vi "Get KB Name.vi"(11 "KB Name":string) -> (3 "KB Name":string)   [LabVIEW 2023, in "LabVIEW RAG.lvlib"]
uses:
  LabVIEW RAG.lvlib
  AI RAG Globals.vi
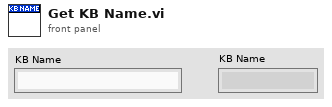
[diagram p1: front panel]
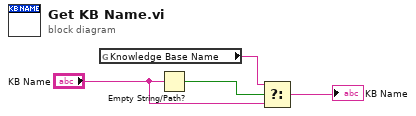
[diagram p0: block diagram]
diagram:
  n1 = global read "AI RAG Globals.vi" "Knowledge Base Name"() -> (w4:string)
  n2 = Empty String/Path?(string/path="KB Name") -> (empty?=w3:bool)
  n3 = Select(t=w4, s=w3, f="KB Name") -> (s? t:f=→"KB Name":string)
